vi "Method.vi"(4 "Value":refnum<class "Abs_Extended Float.lvclass">) -> (1 "Result":refnum<class "Abs_Extended Float.lvclass">)   [LabVIEW 2021, in "Decrement_EXT.lvclass"]
uses:
  Decrement_EXT.lvclass
  Abs_Types/Extended Float/Abs_Extended Float.lvclass
  C:/Users/Tim/Documents/LabVIEW/2021/Data Classes/Source/Functions/Support/One Terminal/EXT/AbsFunc_One Term_EXT.lvclass
  C:/Users/Tim/Documents/LabVIEW/2021/Data Classes/Source/Abs_Types/Extended Float/Abs_Extended Float.lvclass
  Support/One Terminal/EXT/AbsFunc_One Term_EXT.lvclass/AbsFunc_One Term_EXT.ctl
  Support/One Terminal/EXT/Properties/Write Numeric A.vi
  Decrement_EXT.lvclass/Decrement_EXT.ctl
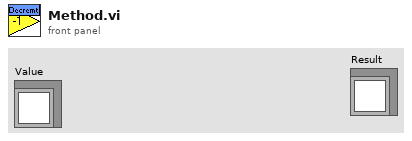
[diagram p1: front panel]
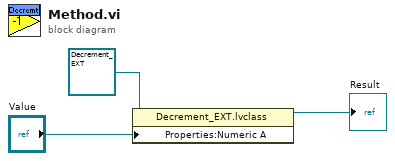
[diagram p0: block diagram]
diagram:
  n1 = property class="Decrement_EXT.lvclass"(reference=refnum<class "Decrement_EXT.lvclass"> refnum ("Decrement_DBL.lvclass"), "Properties:Numeric A"="Value") -> (reference out=→"Result":refnum<class "Decrement_EXT.lvclass">)  [unwired: 1 in, 1 out]
